vi "通信.vi"(8 "error in (no error)":errorcluster, 10 "Slave ID":u8=1, 11 "MB session in":refnum<class "MB_Master.lvclass">) -> (0 "error out":errorcluster, 2 "读取值":T1, 3 "MB session out":refnum<class "MB_Master.lvclass">)   [LabVIEW 2016, in "流量计集成.lvlib" / "LS-H600流量计.lvlib"]
uses:
  <vilib>/Plasmionique/MB Master/MB_Master/MB_Master.lvclass
  <vilib>/Plasmionique/MB Master/MB Master.lvlib
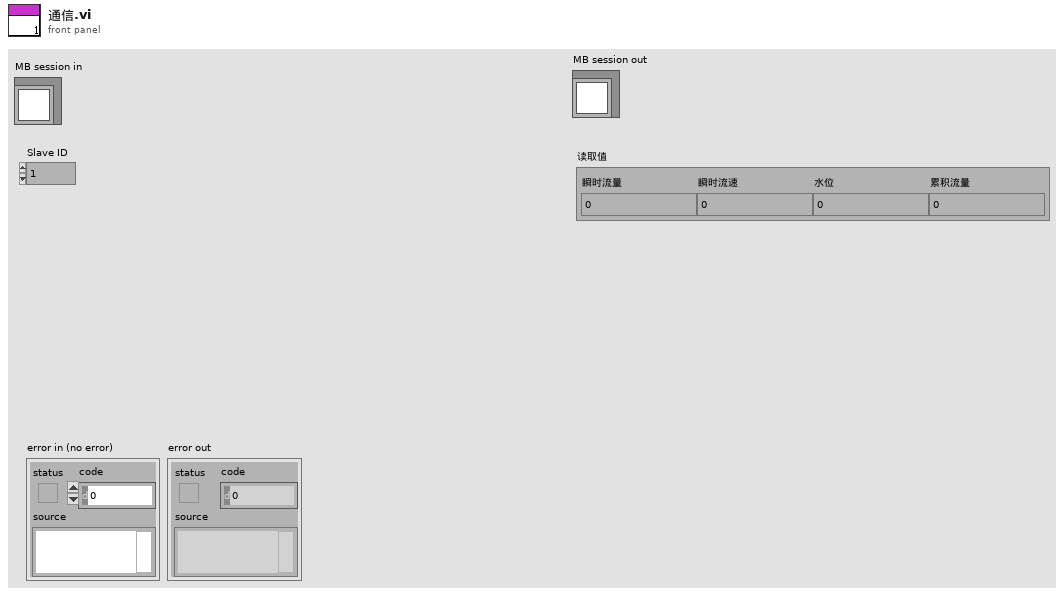
[diagram p1: front panel]
types:
  T1 = typedef "流量计集成.lvlib/LS-H600流量计.lvlib/读取值.ctl" = cluster{"瞬时流量":sgl, "瞬时流速":sgl, "水位":sgl, "累积流量":i32}
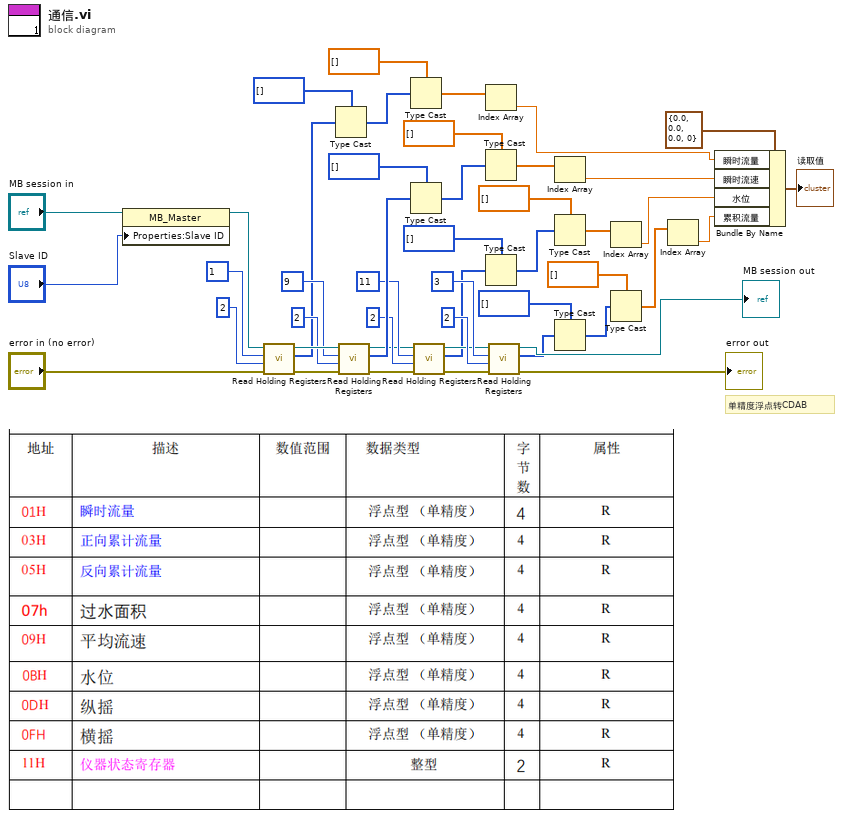
[diagram p0: block diagram]
diagram:
  # "单精度浮点转CDAB"
  n1 = property class="MB_Master"(reference="MB session in", "Properties:Slave ID"="Slave ID") -> (reference out=w40:refnum<class "MB_Master.lvclass">)  [unwired: 1 in, 1 out]
  n2 = call <vilib>:"Read Holding Registers.vi"("error in (no error)"="error in (no error)", "quantity"=u16 2, "starting address"=u16 1, "MB session in"=w40) -> ("error out"=w44:errorcluster, "Registers"=w28:u16[], "MB session out"=w45:refnum<class "MB_Master.lvclass">)  [unwired: 5 in]
  n3 = Type Cast(type=u32[] [], x=w28) -> (*(type *) &x=w21:u32[])
  n4 = call <vilib>:"Read Holding Registers.vi"("error in (no error)"=w44, "quantity"=u16 2, "starting address"=u16 9, "MB session in"=w45) -> ("error out"=w15:errorcluster, "Registers"=w23:u16[], "MB session out"=w16:refnum<class "MB_Master.lvclass">)  [unwired: 5 in]
  n5 = Type Cast(type=sgl[] [], x=w21) -> (*(type *) &x=w27:sgl[])
  n6 = Type Cast(type=u32[] [], x=w23) -> (*(type *) &x=w19:u32[])
  n7 = call <vilib>:"Read Holding Registers.vi"("error in (no error)"=w15, "quantity"=u16 2, "starting address"=u16 11, "MB session in"=w16) -> ("error out"=w13:errorcluster, "Registers"=w8:u16[], "MB session out"=w14:refnum<class "MB_Master.lvclass">)  [unwired: 5 in]
  n8 = Index Array(array=w27) -> (element=w20:sgl)  [unwired: 1 in]
  n9 = Type Cast(type=sgl[] [], x=w19) -> (*(type *) &x=w26:sgl[])
  n10 = Type Cast(type=u32[] [], x=w8) -> (*(type *) &x=w12:u32[])
  n11 = call <vilib>:"Read Holding Registers.vi"("error in (no error)"=w13, "quantity"=u16 2, "starting address"=u16 3, "MB session in"=w14) -> ("error out"=→"error out":errorcluster, "Registers"=w2:u16[], "MB session out"=→"MB session out":refnum<class "MB_Master.lvclass">)  [unwired: 5 in]
  n12 = Index Array(array=w26) -> (element=w22:sgl)  [unwired: 1 in]
  n13 = Type Cast(type=sgl[] [], x=w12) -> (*(type *) &x=w11:sgl[])
  n14 = Type Cast(type=u32[] [], x=w2) -> (*(type *) &x=w3:u32[])
  n15 = Index Array(array=w11) -> (element=w7:sgl)  [unwired: 1 in]
  n16 = Type Cast(type=sgl[] [], x=w3) -> (*(type *) &x=w4:sgl[])
  n17 = Index Array(array=w4) -> (element=w1:sgl)  [unwired: 1 in]
  n18 = Bundle By Name(cluster=T1 {"瞬时流量"=0.0, "瞬时流速"=0.0, "水位"=0.0, "累积流量"=0} ("读取值"), "瞬时流量"=w20, "瞬时流速"=w22, "水位"=w7, "累积流量"=w1) -> (→"读取值":T1)
